vi "Set IPS Action.vi"(8 "error in (no error)":errorcluster, 10 "PSU Act Stat":T1="HOLD" caption="PSU Action Status", 11 "Instrument.Oxford1820 in":refnum<class "Instrument.Oxford1820.lvclass">) -> (0 "error out":errorcluster, 2 "Response":string, 3 "Instrument.Oxford1820 out":refnum<class "Instrument.Oxford1820.lvclass">)   [LabVIEW 2016, in "Instrument.Oxford1820.lvclass"]
uses:
  Instrument.Oxford1820.lvclass
  <instrlib>/Mercury iXX/Public/Libraries/Magnet/Controls/PSU Actions.ctl
  Instrument.Oxford1820.lvclass/Instrument.Oxford1820.ctl
  <instrlib>/Mercury iXX/Public/Libraries/Magnet/Open/Open Magnet Device.vi
  <instrlib>/Mercury iXX/Public/Libraries/Magnet/Configuration/Set/PSU Action Status (Set).vi
  <instrlib>/Mercury iXX/Mercury iXX.lvlib
  <instrlib>/Mercury iXX/Public/Libraries/Magnet.lvlib
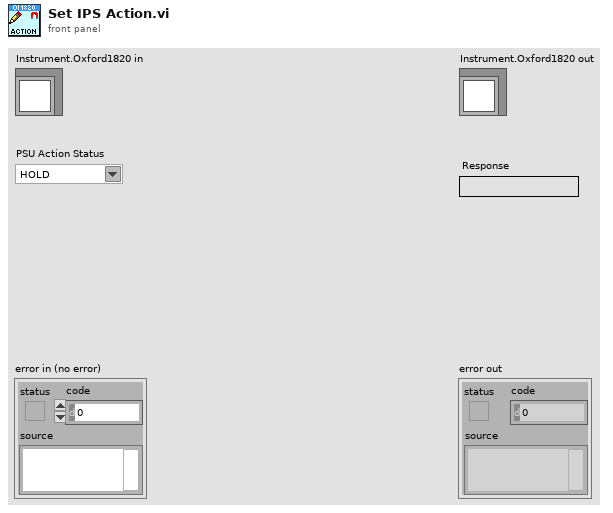
[diagram p1: front panel]
types:
  T1 = typedef "Mercury iXX.lvlib/Magnet.lvlib/PSU Actions.ctl" = string
  T2 = typedef "Mercury iXX.lvlib/Mercury Reference.ctl" = cluster{"Comms":refnum<visa-resource-name>, "Device ID":string[], "Comms Layer":T3, "Command":string, "Query reference":T4}
  T3 = typedef "Mercury iXX.lvlib/Comms Transport Layer.ctl" = enum16{"Ethernet TCP/IP", "USB", "ISOBus - RS-232", "GPIB"}
  T4 = typedef "Mercury iXX.lvlib/Query Dynamic Reference.ctl" = refnum<vi>
  T5 = typedef "Mercury iXX.lvlib/Response String.ctl" = string
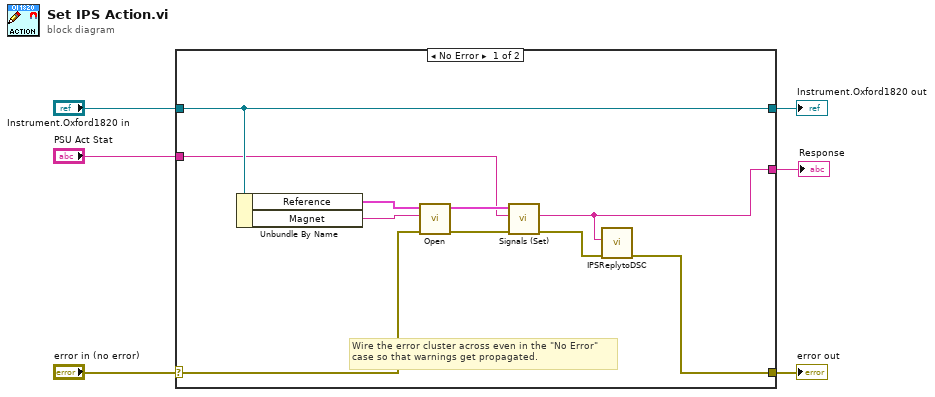
[diagram p0: block diagram]
diagram:
  n1 = case shown="No Error" "error in (no error)" {
    selector: "error in (no error)" -> [w13 w18]
    tunnel: [w7 w18] -> w5
    tunnel: [w16 w17] -> w3
    tunnel: "Instrument.Oxford1820 in" -> [w16 w17]
    tunnel: [w9 _] -> w2
    tunnel: "PSU Act Stat" -> [w10 _]
    frame No Error {
      # "Wire the error cluster across even in the \"No Error\"\ncase so that warnings get propagated."
      n2 = Unbundle By Name(w16) -> ("Reference"=w14:T2, "Magnet"=w15:string)
      n3 = call-poly <instrlib>:"Open.vi"("error in (no error)"=w13, "Device Identifier"=w15, "Mercury Reference In"=w14) -> ("error out"=w11:errorcluster, "Mercury Reference Out"=w12:T2)  [unwired: 7 out]
      n4 = call-poly <instrlib>:"Signals (Set).vi"("error in"=w11, "PSU Act Stat"=w10, "Mercury Reference In"=w12) -> ("error out"=w8:errorcluster, "Response"=w9:T5)  [unwired: 1 in, 6 out]
      n5 = call "IPSReplytoDSC.vi"("error in (no error)"=w8, "Response"=w9) -> ("error out"=w7:errorcluster)  [unwired: 9 in]
    }
    frame Error {
    }
  }
  "error out" <- w5
  "Instrument.Oxford1820 out" <- w3
  "Response" <- w2
